vi "camera_control.vi"() -> ()   [LabVIEW 2011]
uses:
  <vilib>/vision/driver/NI_Vision_Acquisition_Software.lvlib
  <vilib>/userdefined/High Color/IMAQdx.ctl
  <vilib>/vision/NI_Vision_Development_Module.lvlib
  global_vars.vi
panel:
  out "Source Image":u8[][](graph)
  out "Image Pixels (U8)":u8[][][](array[numeric])
  out "Image":T1(plugin-control)
  out "ID_Camera In Use":T2
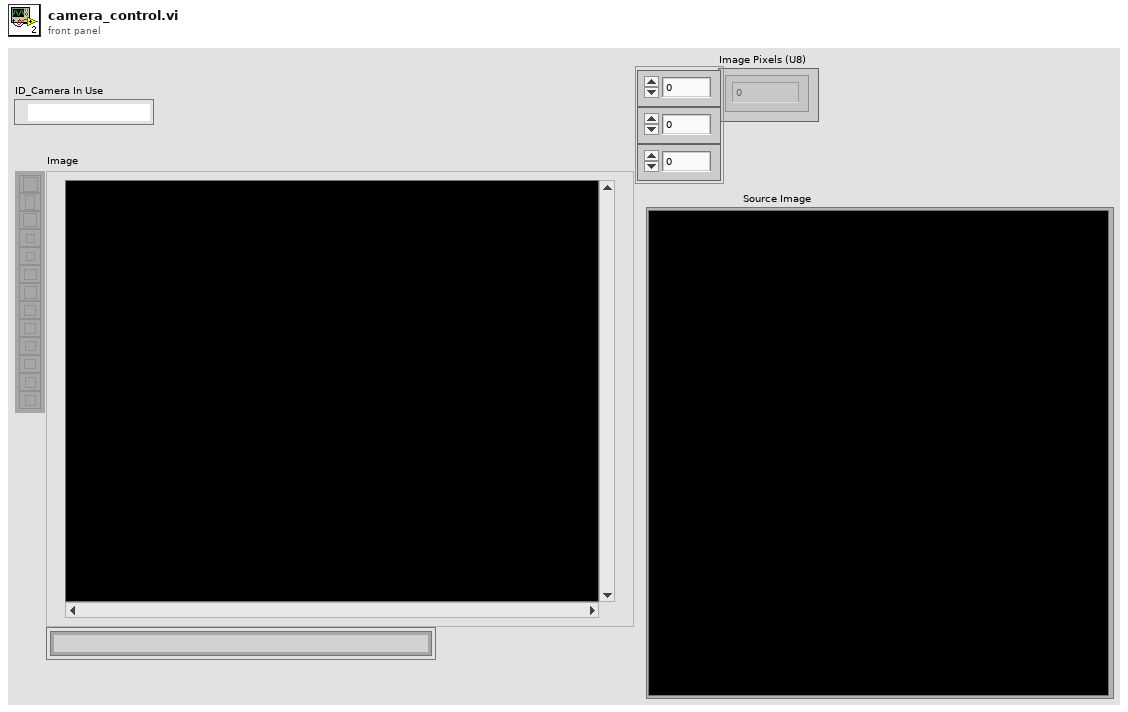
[diagram p1: front panel]
types:
  T1 = typedef "IMAQ Image.ctl" = refnum<image>
  T2 = typedef "IMAQdx.ctl" = refnum<k21>
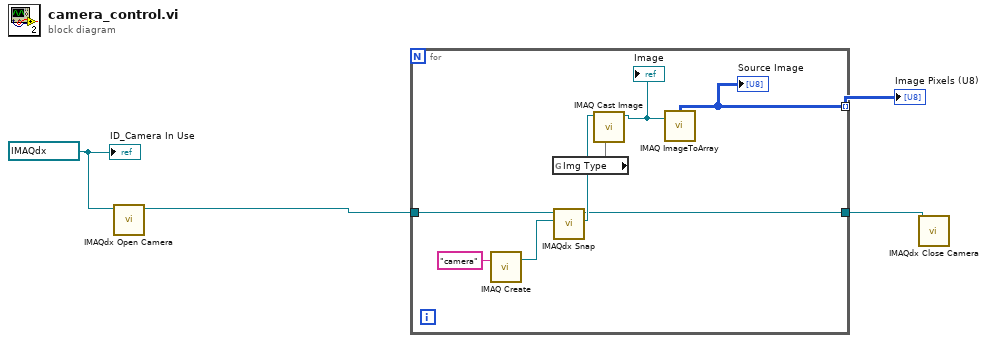
[diagram p0: block diagram]
diagram:
  w4 = T2 "PixeLink" ("ID_Camera")
  n1 = call <vilib>:"IMAQdx Open Camera.vi"("Session In"=w4) -> ("Session Out"=w3:T2)  [unwired: 9 in, 1 out]
  n2 = for {
    tunnel: w3 -> [w8]
    tunnel: [w6] -> w2
    tunnel: [w5] -> w1 mode=indexing
    n3 = call "IMAQ Create"("Image Name"="camera") -> ("New Image"=w12:T1)  [unwired: 3 in, 2 out]
    n4 = global read "global_vars.vi" "Img Type"() -> (w9)
    n5 = call <vilib>:"IMAQdx Snap.vi"("Image In"=w12, "Session In"=w8) -> ("Image Out"=w10:T1, "Session Out"=w6:T2)  [unwired: 7 in, 1 out]
    n6 = call "IMAQ Cast Image"("Image Type"=w9, "Image Src"=w10) -> ("Image Dst Out"=w7:T1)  [unwired: 8 in, 1 out]
    "Image" <- w7
    n7 = call "IMAQ ImageToArray"("Image"=w7) -> ("Image Pixels (U8)"=w5:u8[][])  [unwired: 3 in, 4 out]
    "Source Image" <- w5
  }
  "Image Pixels (U8)" <- w1
  n8 = call <vilib>:"IMAQdx Close Camera.vi"("Session In"=w2) -> ()  [unwired: 10 in, 1 out]
  "ID_Camera In Use" <- w4
